vi "GetTerms4.vi"(0 "XRef":T12, 1 "State In":T10) -> (14 "Terms":T2, 15 "Fatal Error Out":T1)   [LabVIEW 2021, in "FirstXNode .xnode"]
uses:
  FirstXNode .xnode
  <vilib>/XNodeSupport/XNodeXNodeRef.ctl
  State.ctl
  <vilib>/XNodeSupport/XNodeBounds.ctl
  <vilib>/XNodeSupport/XNodeInt.ctl
  <vilib>/XNodeSupport/XNodeTerm4Array.ctl
  <vilib>/XNodeSupport/XNodeTerm4.ctl
  <vilib>/XNodeSupport/XNodeString.ctl
  <vilib>/XNodeSupport/XNodeVariant.ctl
  <vilib>/XNodeSupport/XNodeRect32.ctl
  <vilib>/XNodeSupport/XNodeBool.ctl
  <vilib>/XNodeSupport/XNodeTermDirection.ctl
  <vilib>/XNodeSupport/XNodeErrorCluster.ctl
  <vilib>/XNodeSupport/NI_XNodeSupport.lvlib
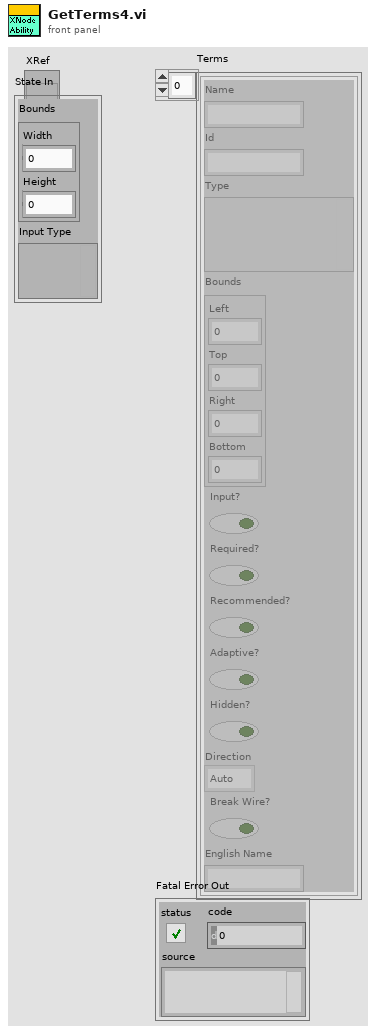
[diagram p1: front panel]
types:
  T1 = typedef "NI_XNodeSupport.lvlib/XNodeErrorCluster.ctl" = errorcluster
  T2 = typedef "NI_XNodeSupport.lvlib/XNodeTerm4Array.ctl" = T3[]
  T3 = typedef "NI_XNodeSupport.lvlib/XNodeTerm4.ctl" = cluster{"Name":T4, "Id":T4, "Type":T5, "Bounds":T6, "Input?":T8, "Required?":T8, "Recommended?":T8, "Adaptive?":T8, "Hidden?":T8, "Direction":T9, "Break Wire?":T8, "English Name":T4}
  T4 = typedef "NI_XNodeSupport.lvlib/XNodeString.ctl" = string
  T5 = typedef "NI_XNodeSupport.lvlib/XNodeVariant.ctl" = variant
  T6 = typedef "NI_XNodeSupport.lvlib/XNodeRect32.ctl" = cluster{"Left":T7, "Top":T7, "Right":T7, "Bottom":T7}
  T7 = typedef "NI_XNodeSupport.lvlib/XNodeInt.ctl" = i32
  T8 = typedef "NI_XNodeSupport.lvlib/XNodeBool.ctl" = bool
  T9 = typedef "NI_XNodeSupport.lvlib/XNodeTermDirection.ctl" = enum32{"Auto", "Up", "Down", "Left", "Right", "Center"}
  T10 = typedef "FirstXNode .xnode/State.ctl" = cluster{"Bounds":T11, "Input Type":variant}
  T11 = typedef "NI_XNodeSupport.lvlib/XNodeBounds.ctl" = cluster{"Width":T7, "Height":T7}
  T12 = typedef "NI_XNodeSupport.lvlib/XNodeXNodeRef.ctl" = refnum<vi>
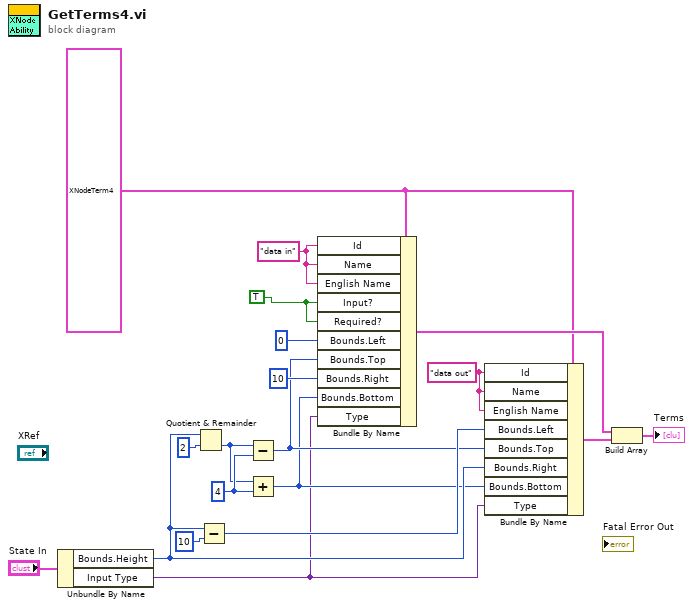
[diagram p0: block diagram]
diagram:
  w1 = "data out"
  w3 = "data in"
  w4 = TRUE
  w17 = T7 4 ("y")
  w2 = T3 {"Name"="", "Id"="", "Type"=variant, "Bounds"={"Left"=0, "Top"=0, "Right"=0, "Bottom"=0}, "Input?"=FALSE, "Required?"=FALSE, "Recommended?"=FALSE, "Adaptive?"=FALSE, "Hidden?"=FALSE, "Direction"=enum."Auto", "Break Wire?"=FALSE, "English Name"=""} ("Term 4")
  n1 = Unbundle By Name("State In") -> ("Bounds.Height"=w11:T7, "Input Type"=w5:variant)
  n2 = Quotient & Remainder(x=w11, y=T7 2) -> (floor(x/y)=w12:T7)  [unwired: 1 out]
  n3 = Subtract(x=w11, y=T7 10 ("Bounds.Right")) -> (x-y=w9:T7)
  n4 = Subtract(x=w12, y=w17) -> (x-y=w8:T7)
  n5 = Add(x=w12, y=w17) -> (x+y=w7:T7)
  n6 = Bundle By Name(cluster=w2, "Id"=w3, "Name"=w3, "English Name"=w3, "Input?"=w4, "Required?"=w4, "Bounds.Left"=T7 0, "Bounds.Top"=w8, "Bounds.Right"=T7 10, "Bounds.Bottom"=w7, "Type"=w5) -> (w15:T3)
  n7 = Bundle By Name(cluster=w2, "Id"=w1, "Name"=w1, "English Name"=w1, "Bounds.Left"=w9, "Bounds.Top"=w8, "Bounds.Right"=w11, "Bounds.Bottom"=w7, "Type"=w5) -> (w6:T3)
  n8 = Build Array(w15, w6) -> (→"Terms":T3[])
